vi "DynamicPersonality.vi"(6 "Pass State\n(inicial)":bool=TRUE, 7 "Pinned":T1={"Attc"="Auto", "Strk"="Auto", "Def"=[], "Strk 2"="Auto"}, 8 "Modo Teste ?":bool, 9 "Qtd Min p/ Stk":dbl=2.0, 10 "our_goalie_id":dbl, 11 "input cluster":T3={"our_robots"=[], "enemy_robots"=[], "balls"=[], "geometry"={"line_width"=0, "field_length"=0, "field_width"=0, "boundary_width"=0, "referee_width"=0, "goal_width"=0, "goal_depth"=0, "goal_wall_width"=0, "center_circle_radius"=0, "defense_radius"=0, "defense_stretch"=0, "free_kick_from_defense_dist"=0, "penalty_spot_from_field_line_dist"=0, "penalty_line_from_spot_dist"=0}, "IA Judge"={"stage"="", "command"="", "our_goalie_id"=0.0, "enemy_goalie_id"=0.0, "command enum"=enum."Halt", "Time"=enum."Azul"}, "Received Timestamp"=timestamp(0 s since 1904-01-01), "Events"={"Touch"=FALSE, "Ball out"=FALSE, "id touch"=0.0, "Ball out of \nVision"=FALSE, "Ball inside \nGoalie area"=FALSE, "Robot not responding"=FALSE, "Robots responding status"=[1.0, 1.0, 1.0, 1.0, 1.0, 1.0], "Enemy Ball \nPossession"=FALSE, "Pass State"=FALSE, "id end of pass"=0.0, "Kick"=FALSE, "Id ini Possession"=0.0, "Ball Possesion"=FALSE, "Id Possesion"=0.0, "Direct Kick"=FALSE, "2nd Strk Ativo"=FALSE}}) -> (2 "output cluster":T3={"our_robots"=[], "enemy_robots"=[], "balls"=[], "geometry"={"line_width"=0, "field_length"=0, "field_width"=0, "boundary_width"=0, "referee_width"=0, "goal_width"=0, "goal_depth"=0, "goal_wall_width"=0, "center_circle_radius"=0, "defense_radius"=0, "defense_stretch"=0, "free_kick_from_defense_dist"=0, "penalty_spot_from_field_line_dist"=0, "penalty_line_from_spot_dist"=0}, "IA Judge"={"stage"="", "command"="", "our_goalie_id"=0.0, "enemy_goalie_id"=0.0, "command enum"=enum."Halt", "Time"=enum."Azul"}, "Received Timestamp"=timestamp(0 s since 1904-01-01), "Events"={"Touch"=FALSE, "Ball out"=FALSE, "id touch"=0.0, "Ball out of \nVision"=FALSE, "Ball inside \nGoalie area"=FALSE, "Robot not responding"=FALSE, "Robots responding status"=[1.0, 1.0, 1.0, 1.0, 1.0, 1.0], "Enemy Ball \nPossession"=FALSE, "Pass State"=FALSE, "id end of pass"=0.0, "Kick"=FALSE, "Id ini Possession"=0.0, "Ball Possesion"=FALSE, "Id Possesion"=0.0, "Direct Kick"=FALSE, "2nd Strk Ativo"=FALSE}})   [LabVIEW 2017]
uses:
  Core/AI Input.ctl
  Core/AI Robot.ctl
  Intel/Functions Enum.ctl
  Intel/AttackerStates.ctl
  Path Planning/RRT/PathDests.ctl
  Path Planning/RRT/PathDest.ctl
  Core/AI Ball.ctl
  Core/Field Size.ctl
  Core/AI Judge.ctl
  Intel/Command Enum.ctl
  Util/Events/Events.ctl
  Select Personalitys.ctl
  Util/Select Auto None or Robot.ctl
panel:
  out "Id 2nd Striker\nPinned":u32
  out "2nd Striker\nPinned?":bool=TRUE
  out "Dfdr\nPinned?":bool
  out "Strk\nPinned?":bool
  out "Attck\nPinned?":bool
  in  "Ids validos":u32[](array[numeric])=[42, 42, 42, 42, 42, 42, 42]
  out "Maior prioridade de \natacante é o mais\nproximo da bola?":bool
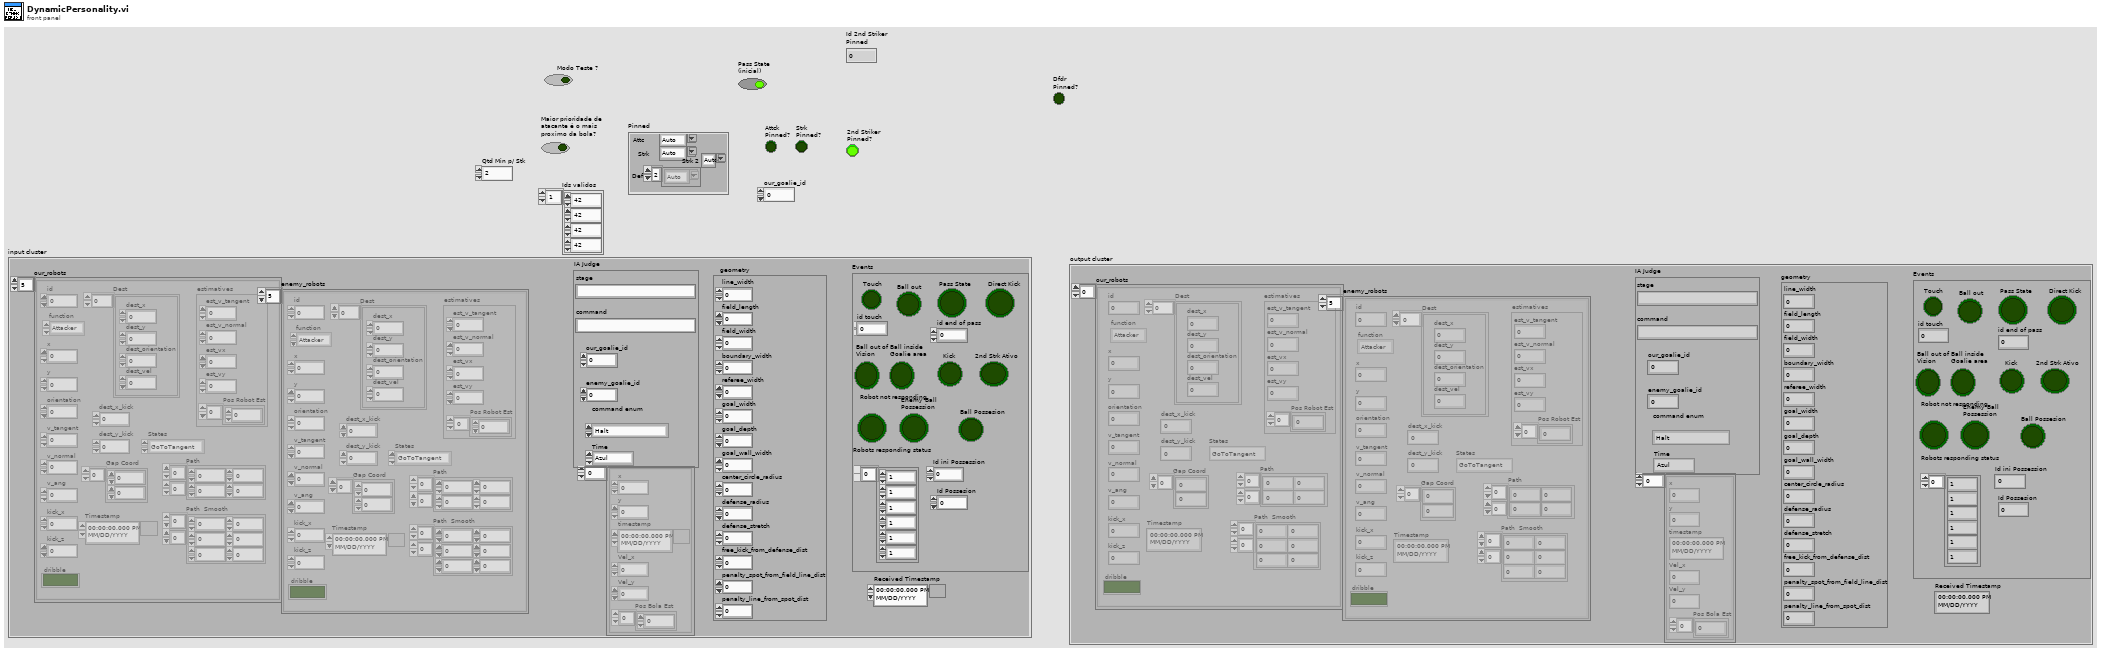
[diagram p1: front panel]
types:
  T1 = typedef "Select Personalitys.ctl" = cluster{"Attc":T2, "Strk":T2, "Def":T2[], "Strk 2":T2}
  T2 = typedef "Select Auto None or Robot.ctl" = string
  T3 = typedef "AI Input.ctl" = cluster{"our_robots":T4[], "enemy_robots":T4[], "balls":T9[], "geometry":T10, "IA Judge":T11, "Received Timestamp":timestamp, "Events":T13}
  T4 = typedef "AI Robot.ctl" = cluster{"id":u32, "function":T5, "x":dbl, "y":dbl, "orientation":dbl, "v_tangent":dbl, "v_normal":dbl, "v_ang":dbl, "kick_x":dbl, "kick_z":dbl, "dribble":bool, "Timestamp":timestamp, "estimatives":cluster{"est_v_tangent":dbl, "est_v_normal":dbl, "est_vx":dbl, "est_vy":dbl, "Pos Robot Est":dbl[]}, "dest_x_kick":dbl, "dest_y_kick":dbl, "Gap Coord":dbl[], "States":T6, "Path ":dbl[][], "Path  Smooth":dbl[][], "Dest":T7}
  T5 = typedef "Functions Enum.ctl" = enum16{"2nd Striker", "Attacker", "Goalie", "Defender", "Striker", "Goto 0", "Dummy", "Kicker", "ZigZag 0", "ZigZag 1", "ZigZag 2", "ZigZag 3", "ZigZag 4", "ZigZag 5", "ZigZag 6", "ZigZag 7", "ZigZag 8", ""}
  T6 = typedef "AttackerStates.ctl" = enum16{"Pass", "GoToTangent", "BallGetting", "GoToKick", ""}
  T7 = typedef "PathDests.ctl" = T8[]
  T8 = typedef "PathDest.ctl" = cluster{"dest_x":dbl, "dest_y":dbl, "dest_orientation":dbl, "dest_vel":dbl}
  T9 = typedef "AI Ball.ctl" = cluster{"x":dbl, "y":dbl, "timestamp":timestamp, "Vel_x":dbl, "Vel_y":dbl, "Pos Bola Est":dbl[]}
  T10 = typedef "Field Size.ctl" = cluster{"line_width":u32, "field_length":u32, "field_width":u32, "boundary_width":u32, "referee_width":u32, "goal_width":u32, "goal_depth":u32, "goal_wall_width":u32, "center_circle_radius":u32, "defense_radius":u32, "defense_stretch":u32, "free_kick_from_defense_dist":u32, "penalty_spot_from_field_line_dist":u32, "penalty_line_from_spot_dist":u32}
  T11 = typedef "AI Judge.ctl" = cluster{"stage":string, "command":string, "our_goalie_id":dbl, "enemy_goalie_id":dbl, "command enum":T12, "Time":enum16{"Azul", "Amarelo"}}
  T12 = typedef "Command Enum.ctl" = enum16{"Halt", "Stop", "Force Start", "PKA Normal Start", "Prepare Kickoff Ally", "PKE Normal Start", "Prepare Kickoff Enemy", "Prepare Penalty Ally", "PPA Normal Start", "Prepare Penalty Enemy", "PPE Normal Start", "Direct Free Enemy", "Direct Free Ally", "Indirect Free Enemy", "Indirect Free Ally", "Timeout Enemy", "Timeout Ally", "Goal Enemy", "Goal Ally", "Ball Placement Enemy", "Ball Placement Ally", "Normal Half Time", "Extra Time Break", "Extra Half Time", "None", "Post Game"}
  T13 = typedef "Events.ctl" = cluster{"Touch":bool, "Ball out":bool, "id touch":dbl, "Ball out of \nVision":bool, "Ball inside \nGoalie area":bool, "Robot not responding":bool, "Robots responding status":dbl[], "Enemy Ball \nPossession":bool, "Pass State":bool, "id end of pass":dbl, "Kick":bool, "Id ini Possession":dbl, "Ball Possesion":bool, "Id Possesion":dbl, "Direct Kick":bool, "2nd Strk Ativo":bool}
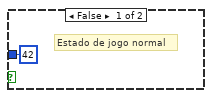
[diagram p4: hidden frame]
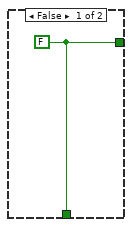
[diagram p9: hidden frame]
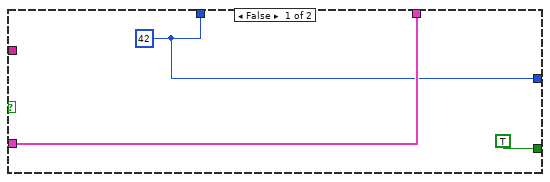
[diagram p11: hidden frame]
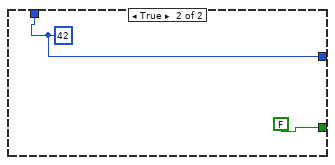
[diagram p13: hidden frame]
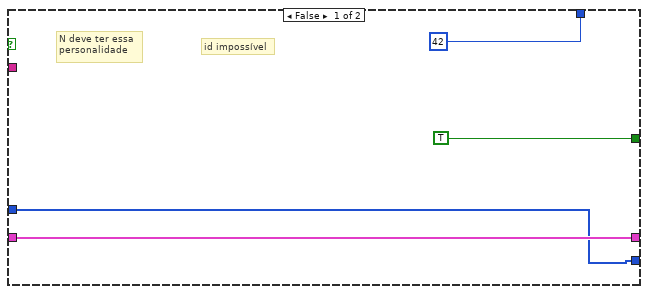
[diagram p17: hidden frame]
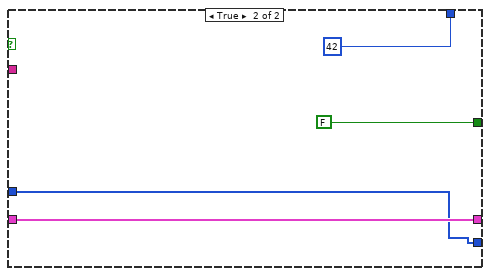
[diagram p19: hidden frame]
diagram:
  # "True: Travado com None\nFalse: Não travado ou travado com id válido"
  # "Descobre id do Striker antes de entrar\nno evento de passe."
  # "personalidades atualizadas"
  # "vai pro feedback node"
  # "personalidades atualizadas"
  # "personalidades atualizadas"
  # "Pinned"
  # "bola parada ?"
  n1 = Unbundle By Name("input cluster") -> ("our_robots"=w148:T4[], "balls"=w105:T9[])
  n2 = Unbundle By Name("Pinned") -> ("Strk"=w149:T2)
  n3 = Not Equal?(x=T2 "None", y=w149) -> (x != y?=w11:bool)
  n4 = case shown="False" w11 {
    tunnel: w149 -> [_ w158]
    tunnel: w148 -> [w153 w157]
    tunnel: [w153 w156] -> w125
    tunnel: [TRUE w155] -> w129
    tunnel: [u32 42 ("Id Maior\nprioridade\natacante") w154] -> w143
    frame False {
      # "id impossível"
      # "N deve ter essa \npersonalidade"
    }
    frame True {
      n5 = Equal?(x=T2 "Auto", y=w158) -> (x = y?=w159:bool)
      n6 = case shown="False" w159 {
        tunnel: w158 -> [w165 _]
        tunnel: w157 -> [w164 w177]
        tunnel: [w163 w177] -> w156
        tunnel: [TRUE FALSE] -> w155
        tunnel: [w161 42] -> w154
        frame False {
          n7 = Decimal String To Number(string=w165) -> (number=w161:i32)  [unwired: 2 in, 1 out]
          n8 = for {
            tunnel: w164 -> [w168] mode=indexing
            tunnel: w161 -> [w169]
            tunnel: [w167] -> w163 mode=indexing
            n9 = Unbundle By Name(w168) -> ("id"=w170:u32)
            n10 = Equal?(x=w169, y=w170) -> (x = y?=w166:bool)
            n11 = case shown="True" w166 {
              tunnel: w168 -> [w171 w174]
              tunnel: [w171 w173] -> w167
              frame False {
              }
              frame True {
                n12 = Bundle By Name(cluster=w174, "function"=Functions_Enum."Striker") -> (w173:T4)
              }
            }
          }
        }
        frame True {
        }
      }
    }
  }
  "Strk\nPinned?" <- w129
  n13 = Unbundle By Name("Pinned") -> ("Def"=w127:T2[])
  n14 = for {
    tunnel: w127 -> [w186] mode=indexing
    tunnel: [w183] -> w123 mode=indexing
    shift-right: [w184] -> w124
    shift-left: w125 -> [w185]
    shift-right: [w181] -> w126
    shift-left: FALSE -> [w182]
    shift-right: [w178] -> _
    shift-left: i32[] [] -> [w179]
    n15 = Not Equal?(x=T2 "None", y=w186) -> (x != y?=w187:bool)
    n16 = case shown="True" w187 {
      tunnel: w186 -> [_ w201]
      tunnel: w185 -> [w192 w200]
      tunnel: [w192 w199] -> w184
      tunnel: [TRUE w198] -> w180
      tunnel: [u32 42 ("Id Maior\nprioridade\natacante") w197] -> w183
      tunnel: w179 -> [w191 w196]
      tunnel: [w191 w195] -> w178
      frame False {
        # "id impossível"
        # "N deve ter essa \npersonalidade"
      }
      frame True {
        n17 = Equal?(x=T2 "Auto", y=w201) -> (x = y?=w202:bool)
        n18 = case shown="False" w202 {
          tunnel: w201 -> [w210 _]
          tunnel: w200 -> [w209 w229]
          tunnel: [w208 w229] -> w199
          tunnel: [TRUE FALSE] -> w198
          tunnel: [w206 42] -> w197
          tunnel: w196 -> [w205 w226]
          tunnel: [w204 w226] -> w195
          frame False {
            n19 = Decimal String To Number(string=w210) -> (number=w206:i32)  [unwired: 2 in, 1 out]
            n20 = for {
              tunnel: w209 -> [w216] mode=indexing
              tunnel: w206 -> [w217]
              tunnel: [w215] -> w208 mode=indexing
              tunnel: w205 -> [w212]
              tunnel: [w211] -> w204
              n21 = Unbundle By Name(w216) -> ("id"=w213:u32)
              n22 = Equal?(x=w217, y=w213) -> (x = y?=w214:bool)
              n23 = case shown="True" w214 {
                tunnel: w216 -> [w219 w225]
                tunnel: [w219 w224] -> w215
                tunnel: w213 -> [_ w221]
                tunnel: w212 -> [w218 w222]
                tunnel: [w218 w220] -> w211
                frame False {
                }
                frame True {
                  n24 = Bundle By Name(cluster=w225, "function"=Functions_Enum."Defender") -> (w224:T4)
                  n25 = Insert Into Array(array=w222, new element=w221) -> (w220:i32[])  [unwired: 1 in]
                }
              }
            }
          }
          frame True {
          }
        }
      }
    }
    n26 = case shown="True" w182 {
      tunnel: [w189 TRUE] -> w181
      tunnel: w180 -> [w189 _]
      frame False {
      }
      frame True {
      }
    }
  }
  "Dfdr\nPinned?" <- w126
  n27 = Unbundle By Name("Pinned") -> ("Attc"=w146:T2)
  n28 = Not Equal?(x=T2 "None", y=w146) -> (x != y?=w145:bool)
  n29 = case shown="True" w145 {
    tunnel: w146 -> [_ w237]
    tunnel: w124 -> [w232 w236]
    tunnel: [w232 w235] -> w50
    tunnel: [TRUE w234] -> w128
    tunnel: [42 w233] -> w144
    frame False {
      # "id impossível"
      # "N deve ter essa \npersonalidade"
    }
    frame True {
      n30 = Equal?(x=T2 "Auto", y=w237) -> (x = y?=w238:bool)
      n31 = case shown="False" w238 {
        tunnel: w237 -> [w244 _]
        tunnel: w236 -> [w243 w256]
        tunnel: [w242 w256] -> w235
        tunnel: [TRUE FALSE] -> w234
        tunnel: [w240 42] -> w233
        frame False {
          n32 = Decimal String To Number(string=w244) -> (number=w240:i32)  [unwired: 2 in, 1 out]
          n33 = for {
            tunnel: w243 -> [w247] mode=indexing
            tunnel: w240 -> [w248]
            tunnel: [w246] -> w242 mode=indexing
            n34 = Unbundle By Name(w247) -> ("id"=w249:u32)
            n35 = Equal?(x=w248, y=w249) -> (x = y?=w245:bool)
            n36 = case shown="True" w245 {
              tunnel: w247 -> [w250 w253]
              tunnel: [w250 w252] -> w246
              frame False {
              }
              frame True {
                n37 = Bundle By Name(cluster=w253, "function"=Functions_Enum."Attacker") -> (w252:T4)
              }
            }
          }
        }
        frame True {
        }
      }
    }
  }
  "Attck\nPinned?" <- w128
  n38 = Unbundle By Name("Pinned") -> ("Strk 2"=w51:T2)
  n39 = Not Equal?(x=w51, y=T2 "None" ("Strk 2")) -> (x != y?=w53:bool)
  n40 = case shown="True" w53 {
    tunnel: [w257 w263] -> w22
    tunnel: [TRUE w262] -> w52
    tunnel: w51 -> [_ w264]
    tunnel: w50 -> [w258 w261]
    tunnel: [w258 w261] -> w41
    tunnel: [w257 w260] -> w21
    frame False {
      w257 = u32 42
    }
    frame True {
      n41 = Equal?(x=w264, y=T2 "Auto" ("Strk 2")) -> (x = y?=w265:bool)
      n42 = case shown="False" w265 {
        tunnel: w264 -> [w271 _]
        tunnel: [w268 w280] -> w263
        tunnel: [TRUE FALSE] -> w262
        tunnel: w261 -> [w269 _]
        tunnel: [w267 w280] -> w260
        frame False {
          n43 = Decimal String To Number(string=w271) -> (number=w268:i32)  [unwired: 2 in, 1 out]
          n44 = for {
            tunnel: w269 -> [w276] mode=indexing
            tunnel: w268 -> [w277]
            shift-right: [w274] -> w267
            shift-left: _ -> [w272]
            n45 = Unbundle By Name(w276) -> ("id"=w273:u32)
            n46 = Equal?(x=w277, y=w273) -> (x = y?=w275:bool)
            n47 = case shown="True" w275 {
              tunnel: [w278 w279] -> w274
              tunnel: w273 -> [_ w279]
              tunnel: w272 -> [w278 _]
              frame False {
              }
              frame True {
              }
            }
          }
        }
        frame True {
          w280 = u32 42
        }
      }
    }
  }
  "2nd Striker\nPinned?" <- w52
  "Id 2nd Striker\nPinned" <- w21
  n48 = for {
    tunnel: w41 -> [w295] mode=indexing
    tunnel: w144 -> [w294]
    tunnel: w143 -> [w293]
    tunnel: w123 -> [w287]
    shift-right: [w290] -> w141
    shift-left: u32[] [] -> [w291]
    tunnel: u32 42 -> [w284]
    # "Deve ter striker?"
    # "Deve ter atacante?"
    n49 = Unbundle By Name(w295) -> ("id"=w283:u32)
    n50 = for {
      tunnel: w283 -> [w298]
      tunnel: [w297] -> w285 mode=indexing
      tunnel: w287 -> [w296] mode=indexing
      n51 = Equal?(x=w296, y=w298) -> (x = y?=w297:bool)
    }
    n52 = Equal?(x=w294, y=w283) -> (x = y?=w292:bool)
    n53 = Equal?(x=w293, y=w283) -> (x = y?=w289:bool)
    n54 = Or Array Elements(Boolean array=w285) -> (logical OR=w286:bool)
    n55 = Equal?(x=w284, y=w283) -> (x = y?=w282:bool)
    n56 = Compound Arithmetic op=OR(w289, w286, w292, w282) -> (w288:bool)
    n57 = case shown="False" w288 {
      tunnel: [w299 w302] -> w290
      tunnel: w291 -> [w301 w302]
      tunnel: w283 -> [w300 _]
      frame False {
        n58 = Insert Into Array(array=w301, new element=w300) -> (w299:u32[])  [unwired: 1 in]
      }
      frame True {
      }
    }
  }
  n59 = Reverse 1D Array(array=w141) -> (reversed array=w139:u32[])
  n60 = for {
    tunnel: w139 -> [w307] mode=indexing
    tunnel: "our_goalie_id" -> [w306]
    shift-right: [w303] -> w60
    shift-left: w139 -> [w305]
    i -> [w304]
    n61 = Equal?(x=w307, y=w306) -> (x = y?=w308:bool)
    n62 = case shown="True" w308 {
      tunnel: w305 -> [w309 w312]
      tunnel: w304 -> [_ w311]
      tunnel: [w309 w310] -> w303
      frame False {
      }
      frame True {
        n63 = Delete From Array(array=w312, index=w311) -> (array with subset deleted=w310:u32[])  [unwired: 1 in, 1 out]
      }
    }
  }
  n64 = Unbundle By Name("input cluster") -> ("Events.Pass State"=w23:bool, "Events.Touch"=w45:bool)
  n65 = case shown="True" w23 {
    tunnel: [u32 42 w314] -> _
    tunnel: w22 -> [_ w314]
    frame False {
      # "Estado de jogo normal"
    }
    frame True {
      # "Evento de passe"
    }
  }
  n66 = Unbundle By Name("input cluster") -> ("balls"=w138:T9[])  [unwired: 1 out]
  n67 = Index Array(array=w138) -> (element=w61:T9)  [unwired: 1 in]
  n68 = for {
    tunnel: w61 -> [w323]
    tunnel: w60 -> [w316] mode=indexing
    tunnel: w41 -> [w326]
    shift-right: [w320] -> w136
    shift-left: dbl[] [] -> [w319]
    shift-right: [w317] -> _
    shift-left: 0.0 -> [w318]
    n69 = while {
      tunnel: w326 -> [w332] mode=indexing
      tunnel: [w331] -> w325
      tunnel: [w330] -> w324
      tunnel: w316 -> [w329]
      tunnel: [w327] -> w315
      stop <- w327 stop-if-true
      n70 = Unbundle By Name(w332) -> ("id"=w328:u32, "x"=w331:dbl, "y"=w330:dbl)
      n71 = Equal?(x=w329, y=w328) -> (x = y?=w327:bool)
    }
    n72 = Unbundle By Name(w323) -> ("x"=w322:dbl, "y"=w321:dbl)
    n73 = case shown="True" w315 {
      tunnel: w325 -> [_ w345]
      tunnel: w324 -> [_ w343]
      tunnel: w322 -> [_ w346]
      tunnel: w321 -> [_ w344]
      tunnel: [w334 w339] -> w320
      tunnel: w319 -> [w334 w338]
      tunnel: w318 -> [w333 w336]
      tunnel: [w333 w335] -> w317
      frame False {
      }
      frame True {
        n74 = Subtract(x=w346, y=w345) -> (x-y=w342:dbl)
        n75 = Subtract(x=w344, y=w343) -> (x-y=w341:dbl)
        n76 = Build Array(w342, w341) -> (w340:dbl[])
        n77 = call "Modulo.vi"("2D vector"=w340) -> ("Modulo"=w337:dbl)  [unwired: 10 in]
        n78 = Insert Into Array(array=w338, index=w336, new element=w337) -> (w339:dbl[])
        n79 = Increment(x=w336) -> (x+1=w335:dbl)
      }
    }
  }
  n80 = feedback #1(FALSE) -> (w46:bool)
  n81 = Index Array(array=w136) -> (element #1=w134:dbl, element #2=w135:dbl)  [unwired: 2 in]
  n82 = feedback #2() -> (w42:bool)  [unwired: 1 in]
  n83 = case shown="True" w23 {
    tunnel: [w347 w350] -> w44
    tunnel: [w347 w349] -> w48
    tunnel: w46 -> [_ w351]
    tunnel: w45 -> [_ w352]
    tunnel: w42 -> [_ w348]
    frame False {
      w347 = FALSE
    }
    frame True {
      n84 = case shown="True" w352 {
        tunnel: [w353 TRUE] -> w349
        tunnel: w351 -> [w353 _]
        frame False {
        }
        frame True {
        }
      }
      n85 = And(x=w348, y=w349) -> (x .and. y?=w350:bool)
    }
  }
  n86 = feedback-in #1(w48) -> ()
  n87 = Less?(x=w134, y=w135) -> (x < y?=w133:bool)
  "Maior prioridade de \natacante é o mais\nproximo da bola?" <- w133
  n88 = Array Size(array=w41) -> (size(s)=w131:i32)
  n89 = local read "Strk\nPinned?"() -> (w58:bool)
  n90 = local read "Attck\nPinned?"() -> (w59:bool)
  n91 = Greater?(x=w131, y=0) -> (0:w132:bool)
  n92 = local read "Id 2nd Striker\nPinned"() -> (w26:u32)
  n93 = local read "2nd Striker\nPinned?"() -> (w28:bool)
  n94 = Equal?(x=w26, y=u32 42) -> (x = y?=w29:bool)
  n95 = And(x=w29, y=w28) -> (x .and. y?=w27:bool)
  n96 = Not Equal?(x=w26, y=u32 42) -> (x != y?=w24:bool)
  n97 = feedback #3() -> (w122:T4[])  [unwired: 1 in]
  n98 = feedback #4(FALSE ("Kick")) -> (w111:bool)
  n99 = Index Array(array=w105) -> (element=w104:T9)  [unwired: 1 in]
  n100 = Unbundle By Name(w104) -> ("Vel_x"=w74:dbl, "Vel_y"=w72:dbl)
  n101 = Absolute Value(x=w72) -> (abs(x)=w71:dbl)
  n102 = Absolute Value(x=w74) -> (abs(x)=w73:dbl)
  n103 = Less Or Equal?(x=w73, y=0.05) -> (x <= y?=w6:bool)
  n104 = Less Or Equal?(x=w71, y=0.05) -> (x <= y?=w5:bool)
  n105 = feedback #5() -> (w2:bool)  [unwired: 1 in]
  n106 = local read "2nd Striker\nPinned?"() -> (w19:bool)
  n107 = local read "Id 2nd Striker\nPinned"() -> (w15:u32)
  n108 = feedback #6() -> (w40:u32)  [unwired: 1 in]
  n109 = feedback #7() -> (w36:u32)  [unwired: 1 in]
  n110 = Not Equal?(x=u32 42, y=w15) -> (x != y?=w18:bool)
  n111 = And(x=w18, y=w19) -> (x .and. y?=w16:bool)
  n112 = feedback #8(FALSE) -> (w116:bool)
  n113 = for {
    tunnel: w41 -> [w384] mode=indexing
    tunnel: w139 -> [w364]
    tunnel: "our_goalie_id" -> [w390]
    tunnel: [w389] -> w35 mode=indexing
    tunnel: w133 -> [w387]
    tunnel: w132 -> [w386]
    tunnel: "input cluster" -> [w385]
    tunnel: w122 -> [w383]
    tunnel: w116 -> [w379]
    tunnel: "input cluster" -> [w371]
    tunnel: [w370] -> w103
    tunnel: [w368] -> _
    tunnel: w41 -> [w367]
    tunnel: w61 -> [w366]
    tunnel: w60 -> [w365]
    tunnel: w59 -> [w363]
    tunnel: w58 -> [w362]
    tunnel: w27 -> [w361]
    tunnel: w44 -> [w360]
    tunnel: [w355] -> w43
    tunnel: w24 -> [w357]
    tunnel: w21 -> [w356]
    tunnel: [w355] -> w3
    i -> [w382]
    n114 = Unbundle By Name(w385) -> ("Events.Pass State"=w377:bool, "IA Judge.command enum"=w368:T12)
    n115 = Unbundle By Name(w384) -> ("id"=w391:u32)
    n116 = for {
      tunnel: w364 -> [w946] mode=indexing
      tunnel: w391 -> [w947]
      shift-right: [w944] -> w388
      shift-left: FALSE -> [w945]
      n117 = Equal?(x=w946, y=w947) -> (x = y?=w943:bool)
      n118 = case shown="True" w943 {
        tunnel: w945 -> [w948 _]
        tunnel: [w948 TRUE] -> w944
        frame False {
        }
        frame True {
        }
      }
    }
    n119 = feedback-in #9(w377) -> ()
    n120 = feedback #9() -> (w378:bool)  [unwired: 1 in]
    n121 = Equal?(x=w377, y=TRUE) -> (x = y?=w373:bool)
    n122 = Equal?(x=w378, y=FALSE) -> (x = y?=w374:bool)
    n123 = And(x=w374, y=w373) -> (x .and. y?=w372:bool)
    n124 = feedback #10() -> (w380:bool)  [unwired: 1 in]
    n125 = case shown="False" w372 {
      selector: w372 -> [_ w405]
      tunnel: [w397 w405] -> w381
      tunnel: w380 -> [w396 _]
      tunnel: w379 -> [w395 _]
      tunnel: [w394 w405] -> w355
      tunnel: w377 -> [w393 _]
      frame False {
        n126 = case shown="True" w395 {
          tunnel: w393 -> [w401 _]
          tunnel: [w398 w404] -> w397
          tunnel: w396 -> [w400 _]
          tunnel: [w399 w404] -> w394
          frame False {
            n127 = case shown="True" w401 {
              selector: w401 -> [w402 _]
              tunnel: w400 -> [_ w403]
              tunnel: [w402 w403] -> w399
              tunnel: [w402 w403] -> w398
              frame False {
              }
              frame True {
              }
            }
          }
          frame True {
            w404 = FALSE
          }
        }
      }
      frame True {
      }
    }
    n128 = feedback-in #10(w381) -> ()
    n129 = Bundle By Name(cluster=w371, "Events.2nd Strk Ativo"="Pass State\n(inicial)", "Events.Pass State"=w355) -> (w370:T3)
    n130 = Unbundle By Name(w370) -> ("Events.Ball out of \nVision"=w369:bool, "Events.2nd Strk Ativo"=w359:bool)
    n131 = case shown="Default" w368 {
      tunnel: w391 -> [w408 w442 w474]
      tunnel: w390 -> [w406 w443 w473]
      tunnel: w384 -> [w410 w446 w472]
      tunnel: [w411 w445 w471] -> w389
      tunnel: w365 -> [w407 _ w470]
      tunnel: w388 -> [w409 _ w469]
      tunnel: w387 -> [_ _ w468]
      tunnel: w386 -> [_ _ w467]
      tunnel: w383 -> [_ _ w456]
      tunnel: w382 -> [_ _ w466]
      tunnel: w355 -> [_ _ _]
      tunnel: w369 -> [_ _ w458]
      tunnel: w367 -> [_ _ w464]
      tunnel: w366 -> [_ _ w463]
      tunnel: w363 -> [_ _ w462]
      tunnel: w362 -> [_ _ w461]
      tunnel: w361 -> [_ _ w460]
      tunnel: w360 -> [_ _ w459]
      tunnel: w359 -> [_ _ w457]
      tunnel: w357 -> [_ _ w455]
      tunnel: w356 -> [_ _ w454]
      tunnel: w355 -> [_ _ w453]
      frame "Prepare Penalty Ally", "PPA Normal Start" {
        # "um atacante, geral defesa"
        n132 = case shown="True" w409 {
          tunnel: [w412 w418] -> w411
          tunnel: w410 -> [w412 w417]
          tunnel: w408 -> [_ w414]
          tunnel: w407 -> [_ w416]
          tunnel: w406 -> [_ w413]
          frame False {
            # "personalidade já definida"
          }
          frame True {
            # "id válido para personalidade dinâmica"
            n133 = Equal?(x=w413, y=w414) -> (x = y?=w415:bool)
            n134 = case shown="False" w415 {
              tunnel: [w423 w440] -> w418
              tunnel: w417 -> [w422 w439]
              tunnel: w414 -> [w420 _]
              tunnel: w416 -> [w419 _]
              frame False {
                # "n é goleiro"
                n135 = local read "Attck\nPinned?"() -> (w421:bool)
                n136 = case shown="True" w421 {
                  tunnel: [w429 w437] -> w423
                  tunnel: w422 -> [w428 w436]
                  tunnel: w420 -> [w426 _]
                  tunnel: w419 -> [w424 _]
                  frame False {
                    # "atacante n definido"
                    n137 = Index Array(array=w424) -> (element=w425:u32)  [unwired: 1 in]
                    n138 = Equal?(x=w426, y=w425) -> (x = y?=w427:bool)
                    n139 = case shown="True" w427 {
                      tunnel: [w431 w434] -> w429
                      tunnel: w428 -> [w430 w433]
                      frame False {
                        # "n é o maior dos ids válidos"
                        n140 = Bundle By Name(cluster=w430, "function"=Functions_Enum."Defender") -> (w431:T4)
                      }
                      frame True {
                        # "maior dos ids válidos"
                        n141 = Bundle By Name(cluster=w433, "function"=Functions_Enum."Attacker") -> (w434:T4)
                      }
                    }
                  }
                  frame True {
                    # "atacante já definido"
                    n142 = Bundle By Name(cluster=w436, "function"=Functions_Enum."Defender") -> (w437:T4)
                  }
                }
              }
              frame True {
                # "é goleiro"
                n143 = Bundle By Name(cluster=w439, "function"=Functions_Enum."Goalie") -> (w440:T4)
              }
            }
          }
        }
      }
      frame "Prepare Penalty Enemy", "PPE Normal Start" {
        # "geral defesa"
        n144 = Equal?(x=w443, y=w442) -> (x = y?=w444:bool)
        n145 = case shown="False" w444 {
          tunnel: w446 -> [w449 w452]
          tunnel: [w448 w451] -> w445
          frame True {
            # "é goleiro"
            n146 = Bundle By Name(cluster=w449, "function"=Functions_Enum."Goalie") -> (w448:T4)
          }
          frame False {
            # "n é goleiro"
            n147 = Bundle By Name(cluster=w452, "function"=Functions_Enum."Defender") -> (w451:T4)
          }
        }
      }
      frame Default {
        n148 = Or(x=w458, y=w457) -> (x .or. y?=w465:bool)
        n149 = case shown="True" w465 {
          tunnel: w474 -> [w484 _]
          tunnel: w473 -> [w483 w623]
          tunnel: w472 -> [w482 w617]
          tunnel: [w481 w626] -> w471
          tunnel: w470 -> [w480 w618]
          tunnel: w469 -> [w479 w625]
          tunnel: w468 -> [w478 _]
          tunnel: w467 -> [w477 w621]
          tunnel: w456 -> [_ w614]
          tunnel: w466 -> [_ w613]
          tunnel: w464 -> [_ w627]
          tunnel: w463 -> [_ w628]
          tunnel: w462 -> [w476 w619]
          tunnel: w461 -> [w475 w620]
          tunnel: w460 -> [_ w622]
          tunnel: w459 -> [_ w615]
          tunnel: w455 -> [_ w612]
          tunnel: w454 -> [_ w611]
          tunnel: w453 -> [_ w610]
          frame False {
            # "estado de jogo normal"
            n150 = case shown="True" w479 {
              tunnel: w484 -> [_ w491]
              tunnel: w483 -> [_ w495]
              tunnel: w482 -> [w485 w493]
              tunnel: [w485 w492] -> w481
              tunnel: w480 -> [_ w490]
              tunnel: w478 -> [_ w489]
              tunnel: w477 -> [_ w488]
              tunnel: w476 -> [_ w487]
              tunnel: w475 -> [_ w486]
              frame False {
                # "Personalidade já definida"
              }
              frame True {
                # "Id válido para personalidade dinâmica"
                n151 = Equal?(x=w495, y=w491) -> (x = y?=w494:bool)
                n152 = case shown="False" w494 {
                  tunnel: w493 -> [w502 w608]
                  tunnel: [w503 w607] -> w492
                  tunnel: w491 -> [w500 _]
                  tunnel: w490 -> [w501 _]
                  tunnel: w489 -> [w499 _]
                  tunnel: w488 -> [w498 _]
                  tunnel: w487 -> [w497 _]
                  tunnel: w486 -> [w496 _]
                  frame False {
                    # "n é goleiro"
                    n153 = Index Array(array=w501) -> (element=w504:u32)  [unwired: 1 in]
                    n154 = Equal?(x=w500, y=w504) -> (x = y?=w505:bool)
                    n155 = case shown="True" w505 {
                      tunnel: [w510 w566] -> w503
                      tunnel: w502 -> [w511 w565]
                      tunnel: w501 -> [w512 _]
                      tunnel: w500 -> [w509 _]
                      tunnel: w499 -> [w507 w564]
                      tunnel: w498 -> [w506 w563]
                      tunnel: w497 -> [_ w562]
                      tunnel: w496 -> [_ w561]
                      frame False {
                        # "n é o maior id dos válidos"
                        n156 = Index Array(array=w512) -> (element #2=w508:u32)  [unwired: 2 in, 1 out]
                        n157 = Equal?(x=w509, y=w508) -> (x = y?=w513:bool)
                        n158 = case shown="True" w513 {
                          tunnel: w511 -> [w514 w520]
                          tunnel: [w515 w519] -> w510
                          tunnel: w507 -> [_ w518]
                          tunnel: w506 -> [_ w517]
                          frame False {
                            # "n é o segundo maior id"
                            n159 = Bundle By Name(cluster=w514, "function"=Functions_Enum."Defender") -> (w515:T4)
                          }
                          frame True {
                            # "segundo maior id"
                            n160 = local read "Strk\nPinned?"() -> (w521:bool)
                            n161 = case shown="False" w521 {
                              tunnel: w520 -> [w525 w553]
                              tunnel: [w526 w552] -> w519
                              tunnel: w518 -> [w523 _]
                              tunnel: w517 -> [w522 _]
                              frame False {
                                # "striker n definido"
                                n162 = local read "Attck\nPinned?"() -> (w524:bool)
                                n163 = case shown="False" w524 {
                                tunnel: [w530 w550] -> w526
                                tunnel: w525 -> [w529 w549]
                                tunnel: w523 -> [w528 _]
                                tunnel: w522 -> [w527 _]
                                frame False {
                                # "attacker ainda n definido"
                                n164 = case shown="True" w528 {
                                tunnel: [w533 w542] -> w530
                                tunnel: w529 -> [w532 w541]
                                tunnel: w527 -> [w531 w540]
                                frame False {
                                # "mais perto da bola"
                                n165 = case shown="True" w531 {
                                tunnel: [w535 w538] -> w533
                                tunnel: w532 -> [w534 w537]
                                frame True {
                                n166 = Bundle By Name(cluster=w534, "function"=Functions_Enum."Attacker") -> (w535:T4)
                                }
                                frame False {
                                n167 = Bundle By Name(cluster=w537, "function"=Functions_Enum."Defender") -> (w538:T4)
                                }
                                }
                                }
                                frame True {
                                # "mais longe da bola"
                                n168 = case shown="False" w540 {
                                tunnel: [w544 w547] -> w542
                                tunnel: w541 -> [w543 w546]
                                frame True {
                                n169 = Bundle By Name(cluster=w543, "function"=Functions_Enum."Striker") -> (w544:T4)
                                }
                                frame False {
                                n170 = Bundle By Name(cluster=w546, "function"=Functions_Enum."Defender") -> (w547:T4)
                                }
                                }
                                }
                                }
                                }
                                frame True {
                                # "attacker travado"
                                n171 = Bundle By Name(cluster=w549, "function"=Functions_Enum."Defender") -> (w550:T4)
                                }
                                }
                              }
                              frame True {
                                # "striker travado"
                                n172 = local read "Attck\nPinned?"() -> (w554:bool)
                                n173 = case shown="False" w554 {
                                tunnel: w553 -> [w555 w558]
                                tunnel: [w556 w559] -> w552
                                frame False {
                                # "atacante n definido"
                                n174 = Bundle By Name(cluster=w555, "function"=Functions_Enum."Defender") -> (w556:T4)
                                }
                                frame True {
                                # "atacante travado"
                                n175 = Bundle By Name(cluster=w558, "function"=Functions_Enum."Defender") -> (w559:T4)
                                }
                                }
                              }
                            }
                          }
                        }
                      }
                      frame True {
                        # "maior id dos válidos"
                        n176 = case shown="True" w562 {
                          tunnel: [w571 w593] -> w566
                          tunnel: w565 -> [w570 w592]
                          tunnel: w564 -> [w569 _]
                          tunnel: w563 -> [w568 w591]
                          tunnel: w561 -> [w567 _]
                          frame False {
                            # "Atacante ainda n definido"
                            n177 = case shown="True" w569 {
                              tunnel: [w575 w589] -> w571
                              tunnel: w570 -> [w574 w588]
                              tunnel: w568 -> [w573 _]
                              tunnel: w567 -> [w572 _]
                              frame False {
                                # "n é o mais perto da bola"
                                n178 = case shown="True" w572 {
                                tunnel: [w578 w586] -> w575
                                tunnel: w574 -> [w577 w585]
                                tunnel: w573 -> [w576 _]
                                frame False {
                                n179 = case shown="False" w576 {
                                tunnel: [w580 w583] -> w578
                                tunnel: w577 -> [w579 w582]
                                frame True {
                                n180 = Bundle By Name(cluster=w579, "function"=Functions_Enum."Striker") -> (w580:T4)
                                }
                                frame False {
                                n181 = Bundle By Name(cluster=w582, "function"=Functions_Enum."Attacker") -> (w583:T4)
                                }
                                }
                                }
                                frame True {
                                n182 = Bundle By Name(cluster=w585, "function"=Functions_Enum."Attacker") -> (w586:T4)
                                }
                                }
                              }
                              frame True {
                                # "mais perto da bola"
                                n183 = Bundle By Name(cluster=w588, "function"=Functions_Enum."Attacker") -> (w589:T4)
                              }
                            }
                          }
                          frame True {
                            # "Atacande já travado"
                            n184 = local read "Strk\nPinned?"() -> (w594:bool)
                            n185 = case shown="False" w594 {
                              tunnel: [w597 w605] -> w593
                              tunnel: w592 -> [w596 w604]
                              tunnel: w591 -> [w595 _]
                              frame False {
                                # "Striker ainda n definido"
                                n186 = case shown="False" w595 {
                                tunnel: [w599 w602] -> w597
                                tunnel: w596 -> [w598 w601]
                                frame True {
                                n187 = Bundle By Name(cluster=w598, "function"=Functions_Enum."Striker") -> (w599:T4)
                                }
                                frame False {
                                n188 = Bundle By Name(cluster=w601, "function"=Functions_Enum."Defender") -> (w602:T4)
                                }
                                }
                              }
                              frame True {
                                # "Sobra defesa"
                                # "Striker já travado"
                                n189 = Bundle By Name(cluster=w604, "function"=Functions_Enum."Defender") -> (w605:T4)
                              }
                            }
                          }
                        }
                      }
                    }
                  }
                  frame True {
                    # "é goleiro"
                    n190 = Bundle By Name(cluster=w608, "function"=Functions_Enum."Goalie") -> (w607:T4)
                  }
                }
              }
            }
          }
          frame True {
            # "2nd Striker Ativo"
            n191 = case shown="False" w615 {
              tunnel: w628 -> [w651 _]
              tunnel: w627 -> [w650 _]
              tunnel: w625 -> [w646 _]
              tunnel: w617 -> [w645 _]
              tunnel: [w644 w938] -> w624
              tunnel: w623 -> [w642 _]
              tunnel: w622 -> [w639 _]
              tunnel: w621 -> [w638 _]
              tunnel: w620 -> [w637 _]
              tunnel: w619 -> [w636 _]
              tunnel: w618 -> [w634 _]
              tunnel: w617 -> [w633 w942]
              tunnel: [w633 w942] -> w616
              tunnel: w614 -> [_ w941]
              tunnel: w613 -> [_ w940]
              tunnel: w612 -> [w632 _]
              tunnel: w611 -> [w631 _]
              tunnel: w610 -> [w629 _]
              frame False {
                (unwired) 5 ("y")
                w649 = inf
                # "Após ter iniciado o evento passe,\nattacker ainda não tocou a bola\n                        OU\nAttacker já tocou a bola e já \nacabou pass state."
                n192 = Array Size(array=w650) -> (size(s)=w647:i32)
                n193 = Greater Or Equal?(x=w647, y=0) -> (x >= y?=w641:bool)
                n194 = Build Array(w649, w649) -> (w648:dbl[])
                n195 = Unbundle By Name(w645) -> ("id"=w643:u32)
                n196 = for {
                  tunnel: w650 -> [w908] mode=indexing
                  tunnel: w651 -> [w902]
                  shift-right: [w898] -> w640
                  shift-left: w648 -> [w899]
                  tunnel: w642 -> [w903]
                  tunnel: w634 -> [w897]
                  n197 = Unbundle By Name(w908) -> ("id"=w896:u32, "x"=w907:dbl, "y"=w906:dbl)
                  n198 = Unbundle By Name(w902) -> ("x"=w905:dbl, "y"=w904:dbl)
                  n199 = for {
                    tunnel: w897 -> [w913] mode=indexing
                    tunnel: w896 -> [w912]
                    shift-right: [w910] -> w894
                    shift-left: FALSE -> [w909]
                    n200 = Equal?(x=w913, y=w912) -> (x = y?=w911:bool)
                    n201 = case shown="True" w909 {
                      tunnel: [w914 TRUE] -> w910
                      tunnel: w911 -> [w914 _]
                      frame False {
                      }
                      frame True {
                      }
                    }
                  }
                  n202 = Build Array(w907, w906) -> (w900:dbl[])
                  n203 = Build Array(w905, w904) -> (w901:dbl[])
                  n204 = case shown="True" w894 {
                    tunnel: w903 -> [_ w923]
                    tunnel: w901 -> [_ w921]
                    tunnel: w900 -> [_ w920]
                    tunnel: w899 -> [w916 w919]
                    tunnel: [w916 w918] -> w898
                    tunnel: w896 -> [_ w917]
                    frame False {
                      # "Robô que está passadno\nno código é um dos fixados\nno pinned"
                    }
                    frame True {
                      # "Robô que está passando\nno código é um dos permitidos\np/ personalidade dinâmica"
                      n205 = Equal?(x=w917, y=w923) -> (x = y?=w922:bool)
                      n206 = case shown="False" w922 {
                        tunnel: w921 -> [w932 _]
                        tunnel: w920 -> [w931 _]
                        tunnel: w919 -> [w926 w937]
                        tunnel: w917 -> [w928 _]
                        tunnel: [w927 w937] -> w918
                        frame False {
                          n207 = Subtract(x=w932, y=w931) -> (x-y=w930:dbl[])
                          n208 = Index Array(array=w926) -> (element #2=w924:dbl)  [unwired: 2 in, 1 out]
                          n209 = call "Modulo.vi"("2D vector"=w930) -> ("Modulo"=w925:dbl)  [unwired: 10 in]
                          n210 = Greater?(x=w924, y=w925) -> (0:w929:bool)
                          n211 = case shown="True" w929 {
                            tunnel: w925 -> [_ w936]
                            tunnel: w928 -> [_ w935]
                            tunnel: [w933 w934] -> w927
                            tunnel: w926 -> [w933 _]
                            frame False {
                            }
                            frame True {
                              n212 = Build Array(w935, w936) -> (w934:dbl[])
                            }
                          }
                        }
                        frame True {
                        }
                      }
                    }
                  }
                }
                n213 = case shown="False" w636 {
                  tunnel: w640 -> [w654 _]
                  tunnel: w634 -> [w653 w667]
                  tunnel: [w652 w667] -> w635
                  frame False {
                    # "Attacker ainda não definido"
                    n214 = for {
                      tunnel: w653 -> [w662] mode=indexing
                      tunnel: w654 -> [w661]
                      tunnel: w653 -> [w658]
                      shift-right: [w656] -> w652
                      shift-left: _ -> [w655]
                      i -> [w657]
                      n215 = Index Array(array=w661) -> (element=w660:dbl)  [unwired: 1 in]
                      n216 = Equal?(x=w660, y=w662) -> (x = y?=w659:bool)
                      n217 = case shown="True" w659 {
                        tunnel: w658 -> [_ w666]
                        tunnel: w657 -> [_ w665]
                        tunnel: [w663 w664] -> w656
                        tunnel: w655 -> [w663 _]
                        frame False {
                        }
                        frame True {
                          n218 = Delete From Array(array=w666, index=w665) -> (array with subset deleted=w664:u32[])  [unwired: 1 in, 1 out]
                        }
                      }
                    }
                  }
                  frame True {
                    # "Atacante já travado"
                  }
                }
                n219 = case shown="True" w646 {
                  tunnel: w645 -> [w669 _]
                  tunnel: [w668 w681] -> w644
                  tunnel: w643 -> [_ w677]
                  tunnel: w642 -> [_ w683]
                  tunnel: w636 -> [_ w680]
                  tunnel: w637 -> [_ w679]
                  tunnel: w641 -> [_ w678]
                  tunnel: w635 -> [_ w676]
                  tunnel: w640 -> [_ w674]
                  tunnel: w639 -> [_ w675]
                  tunnel: w638 -> [_ w673]
                  tunnel: w632 -> [_ w672]
                  tunnel: w631 -> [_ w671]
                  tunnel: w629 -> [_ w670]
                  frame False {
                    # "Personalidade já definida"
                    n220 = Unbundle By Name(w669) -> ("function"=w668:T5)
                  }
                  frame True {
                    # "Id válido para personalidade dinâmica"
                    n221 = Equal?(x=w683, y=w677) -> (x = y?=w682:bool)
                    n222 = case shown="False" w682 {
                      tunnel: [w693 Functions_Enum."Goalie" ("function")] -> w681
                      tunnel: w680 -> [w695 _]
                      tunnel: w679 -> [w694 _]
                      tunnel: w678 -> [w692 _]
                      tunnel: w677 -> [w691 _]
                      tunnel: w676 -> [w690 _]
                      tunnel: w675 -> [w689 _]
                      tunnel: w674 -> [w688 _]
                      tunnel: w673 -> [w687 _]
                      tunnel: w672 -> [w686 _]
                      tunnel: w671 -> [w685 _]
                      tunnel: w670 -> [w684 _]
                      frame False {
                        # "Não é goleiro"
                        n223 = case shown="False" w695 {
                          tunnel: w694 -> [w705 w815]
                          tunnel: [w706 w814] -> w693
                          tunnel: w692 -> [w700 w813]
                          tunnel: w691 -> [w704 w812]
                          tunnel: w690 -> [w702 w811]
                          tunnel: w689 -> [w701 w810]
                          tunnel: w688 -> [w703 _]
                          tunnel: w687 -> [w699 w809]
                          tunnel: w686 -> [w698 w808]
                          tunnel: w685 -> [w697 _]
                          tunnel: w684 -> [w696 _]
                          frame False {
                            # "Attacker ainda não definido"
                            n224 = Index Array(array=w703) -> (element=w708:dbl)  [unwired: 1 in]
                            n225 = Equal?(x=w708, y=w704) -> (x = y?=w707:bool)
                            n226 = case shown="False" w707 {
                              tunnel: [w715 Functions_Enum."Attacker" ("function")] -> w706
                              tunnel: w705 -> [w718 _]
                              tunnel: w704 -> [w717 _]
                              tunnel: w702 -> [w716 _]
                              tunnel: w701 -> [w714 _]
                              tunnel: w700 -> [w713 _]
                              tunnel: w699 -> [w712 _]
                              tunnel: w698 -> [w711 _]
                              tunnel: w697 -> [w710 _]
                              tunnel: w696 -> [w709 _]
                              frame False {
                                # "Robô que está passando pelo código NÃO\né o mais próximo à bola"
                                n227 = case shown="True" w712 {
                                tunnel: w718 -> [_ w728]
                                tunnel: w717 -> [_ w727]
                                tunnel: w716 -> [_ w726]
                                tunnel: [Functions_Enum."Defender" ("function") w725] -> w715
                                tunnel: w714 -> [_ w724]
                                tunnel: w713 -> [_ w723]
                                tunnel: w711 -> [_ w722]
                                tunnel: w710 -> [_ w721]
                                tunnel: w709 -> [_ w720]
                                frame False {
                                # "Não qtdade min p/ Striker"
                                }
                                frame True {
                                # "Tem qtdade min p/ Striker"
                                n228 = case shown="False" w728 {
                                tunnel: w727 -> [w733 w779]
                                tunnel: w726 -> [w732 w778]
                                tunnel: [w736 w781] -> w725
                                tunnel: w724 -> [w735 w782]
                                tunnel: w723 -> [w734 w780]
                                tunnel: w722 -> [w731 w777]
                                tunnel: w721 -> [w730 _]
                                tunnel: w720 -> [w729 _]
                                frame False {
                                # "Striker ainda não definido"
                                n229 = Index Array(array=w732) -> (element=w738:u32)  [unwired: 1 in]
                                n230 = Equal?(x=w738, y=w733) -> (x = y?=w737:bool)
                                n231 = case shown="False" w737 {
                                tunnel: [w745 Functions_Enum."Striker" ("function")] -> w736
                                tunnel: w735 -> [w746 _]
                                tunnel: w734 -> [w744 _]
                                tunnel: w733 -> [w743 _]
                                tunnel: w732 -> [w742 _]
                                tunnel: w731 -> [w741 _]
                                tunnel: w730 -> [w740 _]
                                tunnel: w729 -> [w739 _]
                                frame False {
                                # "Robô que está passando pelo código NÃO\né o de maior id dos não fixados"
                                n232 = case shown="False" w746 {
                                tunnel: [w752 Functions_Enum."Defender" ("function")] -> w745
                                tunnel: w744 -> [w751 _]
                                tunnel: w743 -> [w754 _]
                                tunnel: w742 -> [w753 _]
                                tunnel: w741 -> [w749 _]
                                tunnel: w740 -> [w750 _]
                                tunnel: w739 -> [w747 _]
                                frame False {
                                # "Quando termina o Pass\nState, não precisamos \nmais que o 2nd Stiker \nseja o fixado e o código \nescolhe pelo id."
                                # "2nd Striker NÃO fixado ou fixado com id válido"
                                n233 = case shown="False" w747 {
                                selector: w747 -> [w755 _]
                                tunnel: w749 -> [_ w756]
                                tunnel: [w755 w756] -> w748
                                frame False {
                                }
                                frame True {
                                }
                                }
                                n234 = case shown="True" w748 {
                                tunnel: w754 -> [w760 w772]
                                tunnel: w753 -> [w759 _]
                                tunnel: [w758 w770] -> w752
                                tunnel: w751 -> [w757 _]
                                tunnel: w750 -> [_ w769]
                                frame False {
                                # "2nd Striker não fixado"
                                n235 = case shown="True" w757 {
                                tunnel: w760 -> [_ w766]
                                tunnel: w759 -> [_ w764]
                                tunnel: [Functions_Enum."Defender" ("function") w762] -> w758
                                frame False {
                                # "Quantidade de robôs NÃO\nsuficiente p/ ter 2nd Striker.\nSobra ser defender"
                                }
                                frame True {
                                # "Quantidade de robôs \nsuficiente p/ ter 2nd Striker"
                                n236 = Index Array(array=w764) -> (element #2=w765:u32)  [unwired: 2 in, 1 out]
                                n237 = Equal?(x=w765, y=w766) -> (x = y?=w763:bool)
                                n238 = case shown="True" w763 {
                                tunnel: [Functions_Enum."Defender" ("function") Functions_Enum."2nd Striker" ("function")] -> w762
                                frame False {
                                }
                                frame True {
                                # "Robô que está passando pelo código\né o de segundo maior id dos não fixados"
                                }
                                }
                                }
                                }
                                }
                                frame True {
                                # "2nd Striker travado com id válido"
                                n239 = Equal?(x=w769, y=w772) -> (x = y?=w771:bool)
                                n240 = case shown="True" w771 {
                                tunnel: [Functions_Enum."Defender" ("function") Functions_Enum."2nd Striker" ("function")] -> w770
                                frame False {
                                # "Robô que está passando pelo código NÃO é o fixado como 2nd Striker"
                                }
                                frame True {
                                # "Robô que está passando pelo código é o fixado como 2nd Striker"
                                }
                                }
                                }
                                }
                                }
                                frame True {
                                # "2nd Striker fixado com None"
                                }
                                }
                                }
                                frame True {
                                # "Robô que está passando pelo código\né o de maior id dos não fixados"
                                }
                                }
                                }
                                frame True {
                                # "Striker já travado"
                                n241 = case shown="False" w782 {
                                tunnel: [w784 Functions_Enum."Defender" ("function")] -> w781
                                tunnel: w780 -> [w787 _]
                                tunnel: w779 -> [w786 _]
                                tunnel: w778 -> [w785 _]
                                tunnel: w777 -> [w783 _]
                                frame False {
                                # "2nd Striker NÃO fixado ou fixado com id válido"
                                n242 = case shown="False" w783 {
                                tunnel: w787 -> [w791 _]
                                tunnel: w786 -> [w790 w803]
                                tunnel: w785 -> [w789 _]
                                tunnel: [w788 w800] -> w784
                                frame False {
                                # "2nd Striker não fixado"
                                n243 = case shown="True" w791 {
                                tunnel: w790 -> [_ w797]
                                tunnel: w789 -> [_ w795]
                                tunnel: [Functions_Enum."Defender" ("function") w793] -> w788
                                frame False {
                                # "Quantidade de robôs NÃO\nsuficiente p/ ter 2nd Striker"
                                }
                                frame True {
                                # "Quantidade de robôs \nsuficiente p/ ter 2nd Striker"
                                n244 = Index Array(array=w795) -> (element=w796:u32)  [unwired: 1 in]
                                n245 = Equal?(x=w796, y=w797) -> (x = y?=w794:bool)
                                n246 = case shown="False" w794 {
                                tunnel: [Functions_Enum."Defender" ("function") Functions_Enum."2nd Striker" ("function")] -> w793
                                frame False {
                                # "Robô que está passando pelo código NÃO\né o de maior id dos não fixados"
                                }
                                frame True {
                                # "Robô que está passando pelo código\né o de maior id dos não fixados"
                                }
                                }
                                }
                                }
                                }
                                frame True {
                                # "2nd Striker travado com id válido"
                                n247 = local read "Id 2nd Striker\nPinned"() -> (w802:u32)
                                n248 = Equal?(x=w802, y=w803) -> (x = y?=w801:bool)
                                n249 = case shown="False" w801 {
                                tunnel: [Functions_Enum."Defender" ("function") Functions_Enum."2nd Striker" ("function")] -> w800
                                frame False {
                                # "Robô que está passando no código NÃO é o fixado como 2nd Striker"
                                }
                                frame True {
                                # "Robô que está passando no código é o fixado como 2nd Striker"
                                }
                                }
                                }
                                }
                                }
                                frame True {
                                # "2nd Striker fixado com None"
                                }
                                }
                                }
                                }
                                }
                                }
                              }
                              frame True {
                                # "Robô que está passando pelo código\né o mais próximo à bola"
                              }
                            }
                          }
                          frame True {
                            # "Atacante já travado"
                            n250 = case shown="True" w809 {
                              tunnel: w815 -> [_ w823]
                              tunnel: [Functions_Enum."Defender" ("function") w822] -> w814
                              tunnel: w813 -> [_ w821]
                              tunnel: w812 -> [_ w820]
                              tunnel: w811 -> [_ w819]
                              tunnel: w810 -> [_ w818]
                              tunnel: w808 -> [_ w817]
                              frame False {
                                # "NÃO tem qtdade min p/ Striker"
                              }
                              frame True {
                                # "Tem qtdade min p/ Striker"
                                n251 = case shown="False" w823 {
                                tunnel: [w829 w868] -> w822
                                tunnel: w821 -> [w827 w867]
                                tunnel: w820 -> [w826 w866]
                                tunnel: w819 -> [w825 w865]
                                tunnel: w818 -> [w828 w864]
                                tunnel: w817 -> [w824 w863]
                                frame False {
                                # "Striker ainda não definido"
                                n252 = Index Array(array=w825) -> (element=w831:u32)  [unwired: 1 in]
                                n253 = Equal?(x=w831, y=w826) -> (x = y?=w830:bool)
                                n254 = case shown="False" w830 {
                                tunnel: [w836 Functions_Enum."Striker" ("function")] -> w829
                                tunnel: w828 -> [w837 _]
                                tunnel: w827 -> [w835 _]
                                tunnel: w826 -> [w832 _]
                                tunnel: w825 -> [w834 _]
                                tunnel: w824 -> [w833 _]
                                frame False {
                                # "Robô que está passando pelo código NÃO\né o de maior id dos não fixados"
                                n255 = case shown="False" w837 {
                                tunnel: [w838 Functions_Enum."Defender" ("function")] -> w836
                                tunnel: w835 -> [w840 _]
                                tunnel: w832 -> [w842 _]
                                tunnel: w834 -> [w841 _]
                                tunnel: w833 -> [w839 _]
                                frame False {
                                # "2nd Striker NÃO fixado ou fixado com id válido"
                                n256 = case shown="True" w839 {
                                tunnel: w842 -> [w846 w858]
                                tunnel: w841 -> [w845 _]
                                tunnel: w840 -> [w844 _]
                                tunnel: [w843 w855] -> w838
                                frame False {
                                # "2nd Striker não fixado"
                                n257 = case shown="True" w844 {
                                tunnel: w846 -> [_ w852]
                                tunnel: w845 -> [_ w851]
                                tunnel: [Functions_Enum."Defender" ("function") w848] -> w843
                                frame False {
                                # "Quantidade de robôs NÃO\nsuficiente p/ ter 2nd Striker.\nSobra ser defender"
                                }
                                frame True {
                                # "Quantidade de robôs \nsuficiente p/ ter 2nd Striker"
                                n258 = Index Array(array=w851) -> (element #2=w850:u32)  [unwired: 2 in, 1 out]
                                n259 = Equal?(x=w850, y=w852) -> (x = y?=w849:bool)
                                n260 = case shown="False" w849 {
                                tunnel: [Functions_Enum."Defender" ("function") Functions_Enum."2nd Striker" ("function")] -> w848
                                frame False {
                                }
                                frame True {
                                # "Robô que está passando pelo código\né o de segundo maior id dos não fixados"
                                }
                                }
                                }
                                }
                                }
                                frame True {
                                # "2nd Striker fixado com id válido"
                                n261 = local read "Id 2nd Striker\nPinned"() -> (w857:u32)
                                n262 = Equal?(x=w857, y=w858) -> (x = y?=w856:bool)
                                n263 = case shown="True" w856 {
                                tunnel: [Functions_Enum."Defender" ("function") Functions_Enum."2nd Striker" ("function")] -> w855
                                frame False {
                                # "Robô que está passando pelo código NÃO é o 2nd Striker fixado no pinned"
                                }
                                frame True {
                                # "Robô que está passando pelo código é o 2nd Striker fixado no pinned"
                                }
                                }
                                }
                                }
                                }
                                frame True {
                                # "2nd Striker fixado com id inválido (None)"
                                }
                                }
                                }
                                frame True {
                                # "Robô que está passando pelo código\né o de maior id dos não fixados"
                                }
                                }
                                }
                                frame True {
                                # "Striker já travado"
                                n264 = case shown="False" w864 {
                                tunnel: [w872 Functions_Enum."Defender" ("function")] -> w868
                                tunnel: w867 -> [w873 _]
                                tunnel: w866 -> [w871 _]
                                tunnel: w865 -> [w870 _]
                                tunnel: w863 -> [w869 _]
                                frame False {
                                # "2nd Striker não fixado ou fixado com id válido"
                                n265 = case shown="True" w869 {
                                tunnel: w873 -> [w877 _]
                                tunnel: [w876 w886] -> w872
                                tunnel: w871 -> [w875 w889]
                                tunnel: w870 -> [w874 _]
                                frame False {
                                # "2nd Striker não fixado"
                                n266 = case shown="False" w877 {
                                tunnel: [Functions_Enum."Defender" ("function") w879] -> w876
                                tunnel: w875 -> [_ w883]
                                tunnel: w874 -> [_ w882]
                                frame False {
                                # "Quantidade de robôs NÃO\nsuficiente p/ ter 2nd Striker.\nSobra ser defender"
                                }
                                frame True {
                                # "Quantidade de robôs \nsuficiente p/ ter 2nd Striker"
                                n267 = Index Array(array=w882) -> (element=w881:u32)  [unwired: 1 in]
                                n268 = Equal?(x=w881, y=w883) -> (x = y?=w880:bool)
                                n269 = case shown="False" w880 {
                                tunnel: [Functions_Enum."Defender" ("function") Functions_Enum."2nd Striker" ("function")] -> w879
                                frame False {
                                }
                                frame True {
                                # "Robô que está passando pelo código\né o de maior id dos não fixados"
                                }
                                }
                                }
                                }
                                }
                                frame True {
                                # "2nd Striker fixado com id válido"
                                n270 = local read "Id 2nd Striker\nPinned"() -> (w888:u32)
                                n271 = Equal?(x=w888, y=w889) -> (x = y?=w887:bool)
                                n272 = case shown="True" w887 {
                                tunnel: [Functions_Enum."Defender" ("function") Functions_Enum."2nd Striker" ("function")] -> w886
                                frame False {
                                # "Robô que está passando no código NÃO é o robô fixado, no pinned, para ser 2nd Striker"
                                }
                                frame True {
                                # "Robô que está passando no código é o robô fixado, no pinned, para ser 2nd Striker"
                                }
                                }
                                }
                                }
                                }
                                frame True {
                                # "2nd Striker fixado com id inválido (None)"
                                }
                                }
                                }
                                }
                              }
                            }
                          }
                        }
                      }
                      frame True {
                        # "É goleiro"
                      }
                    }
                  }
                }
              }
              frame True {
                # "Após ter iniciado o evento de passe,\nAttacker já tocou a bola mas ainda \nnão acabou o pass state."
                n273 = Index Array(array=w941, index=w940) -> (element=w939:T4)
                n274 = Unbundle By Name(w939) -> ("function"=w938:T5)
              }
            }
            n275 = Bundle By Name(cluster=w616, "function"=w624) -> (w626:T4)
          }
        }
      }
    }
  }
  n276 = feedback-in #2(w43) -> ()
  n277 = feedback-in #3(w35) -> ()
  n278 = Unbundle By Name(w103) -> ("Events.Kick"=w112:bool, "balls"=w121:T9[])
  n279 = for {
    shift-right: [w955] -> w9
    shift-left: _ -> [w953]
    tunnel: w35 -> [w952] mode=indexing
    n280 = Unbundle By Name(w952) -> ("id"=w954:u32, "function"=w951:T5)
    n281 = Equal?(x=w951, y=Functions_Enum."Striker") -> (x = y?=w950:bool)
    n282 = case shown="True" w950 {
      tunnel: [w957 w958] -> w955
      tunnel: w954 -> [_ w958]
      tunnel: w953 -> [w957 _]
      frame False {
      }
      frame True {
      }
    }
  }
  n283 = for {
    tunnel: w35 -> [w965] mode=indexing
    shift-right: [w959] -> w37
    shift-left: u32[] [] -> [w961]
    n284 = Unbundle By Name(w965) -> ("id"=w960:u32, "function"=w964:T5)
    n285 = Equal?(x=w964, y=Functions_Enum."Defender") -> (x = y?=w962:bool)
    n286 = case shown="True" w962 {
      tunnel: w961 -> [w966 w969]
      tunnel: w960 -> [_ w968]
      tunnel: [w966 w967] -> w959
      frame False {
      }
      frame True {
        n287 = Insert Into Array(array=w969, new element=w968) -> (w967:u32[])  [unwired: 1 in]
      }
    }
  }
  n288 = Index Array(array=w121) -> (element=w120:T9)  [unwired: 1 in]
  n289 = Unbundle By Name(w120) -> ("Vel_x"=w110:dbl, "Vel_y"=w109:dbl, "x"=w119:dbl, "y"=w118:dbl)
  n290 = Build Array(w110, w109) -> (w108:dbl[])
  n291 = Build Array(w119, w118) -> (w33:dbl[])
  n292 = case shown="False" w112 {
    selector: w112 -> [_ w979]
    tunnel: [w971 w979] -> w113
    tunnel: w111 -> [w970 _]
    tunnel: w108 -> [w977 _]
    tunnel: [w973 FALSE] -> _
    frame False {
      n293 = call "Modulo.vi"("2D vector"=w977) -> ("Modulo"=w976:dbl)  [unwired: 10 in]
      n294 = Less?(x=w976, y=0.01) -> (x < y?=w974:bool)
      n295 = And(x=w974, y=w970) -> (x .and. y?=w973:bool)
      n296 = Select(t=FALSE ("Kick"), s=w973, f=w970) -> (s? t:f=w971:bool)
    }
    frame True {
    }
  }
  n297 = feedback-in #4(w113) -> ()
  n298 = Array Max & Min(array=w37) -> (max value=w14:u32)  [unwired: 3 out]
  n299 = case shown="False" w11 {
    tunnel: [u32 42 ("id") w981] -> w10
    tunnel: w9 -> [_ w981]
    frame False {
      # "Strk None"
    }
    frame True {
      # "Strk existe"
    }
  }
  n300 = feedback-in #5(w3) -> ()
  n301 = Not Equal?(x=w3, y=w2) -> (x != y?=w1:bool)
  n302 = Not(x=w1) -> (.not. x?=w8:bool)
  n303 = Compound Arithmetic op=AND(w6, w5, w8) -> (w4:bool)
  n304 = Bundle By Name(cluster=w103, "our_robots"=w35) -> (w64:T3)
  n305 = case shown="False" w16 {
    tunnel: w15 -> [_ w983]
    tunnel: [w982 w983] -> w13
    tunnel: w14 -> [w982 _]
    frame False {
    }
    frame True {
      # "2nd Striker pinned com id válido"
    }
  }
  n306 = case shown="True" w23 {
    tunnel: [w985 w987] -> w39
    tunnel: w10 -> [w985 _]
    tunnel: w40 -> [_ w987]
    tunnel: w13 -> [w984 _]
    tunnel: [w984 w986] -> w34
    tunnel: w36 -> [_ w986]
    frame False {
      # "Estado normal"
    }
    frame True {
      # "Estado de passe"
    }
  }
  n307 = for {
    tunnel: w35 -> [w997] mode=indexing
    tunnel: w33 -> [w993]
    shift-right: [w992] -> w107
    shift-left: FALSE -> [w991]
    tunnel: w39 -> [w990]
    n308 = Unbundle By Name(w997) -> ("x"=w996:dbl, "y"=w995:dbl, "id"=w989:u32)
    n309 = Equal?(x=w989, y=w990) -> (x = y?=w988:bool)
    n310 = Build Array(w996, w995) -> (w994:dbl[])
    n311 = case shown="True" w988 {
      tunnel: w994 -> [_ w1003]
      tunnel: w993 -> [_ w1004]
      tunnel: [w998 w999] -> w992
      tunnel: w991 -> [w998 _]
      frame False {
      }
      frame True {
        n312 = Subtract(x=w1004, y=w1003) -> (x-y=w1002:dbl[])
        n313 = call "Modulo.vi"("2D vector"=w1002) -> ("Modulo"=w1001:dbl)  [unwired: 10 in]
        n314 = Less?(x=w1001, y=200.0) -> (x < y?=w999:bool)
      }
    }
  }
  n315 = for {
    tunnel: w35 -> [w1014] mode=indexing
    tunnel: w34 -> [w1012]
    tunnel: w33 -> [w1007]
    shift-right: [w1006] -> w31
    shift-left: FALSE -> [w1005]
    n316 = Unbundle By Name(w1014) -> ("x"=w1010:dbl, "y"=w1009:dbl, "id"=w1013:u32)
    n317 = Equal?(x=w1013, y=w1012) -> (x = y?=w1011:bool)
    n318 = Build Array(w1010, w1009) -> (w1008:dbl[])
    n319 = case shown="True" w1011 {
      tunnel: w1008 -> [_ w1021]
      tunnel: w1007 -> [_ w1020]
      tunnel: [w1015 w1016] -> w1006
      tunnel: w1005 -> [w1015 _]
      frame False {
      }
      frame True {
        n320 = Subtract(x=w1021, y=w1020) -> (x-y=w1019:dbl[])
        n321 = call "Modulo.vi"("2D vector"=w1019) -> ("Modulo"=w1018:dbl)  [unwired: 10 in]
        n322 = Less?(x=w1018, y=200.0) -> (x < y?=w1016:bool)
      }
    }
  }
  n323 = feedback-in #6(w39) -> ()
  n324 = feedback-in #7(w34) -> ()
  n325 = Compound Arithmetic op=OR(w31, FALSE ("value"), w107) -> (w106:bool)
  n326 = feedback-in #8(w106) -> ()
  n327 = feedback #11(w64) -> (w102:T3)
  n328 = case shown="True" w4 {
    tunnel: w102 -> [_ w1028]
    tunnel: [w1022 w1023] -> w96
    tunnel: w64 -> [w1022 w1024]
    frame False {
    }
    frame True {
      n329 = Unbundle By Name(w1024) -> ("our_robots"=w1026:T4[])
      n330 = Unbundle By Name(w1028) -> ("our_robots"=w1027:T4[])
      n331 = for {
        tunnel: w1027 -> [w1031] mode=indexing
        tunnel: w1026 -> [w1032] mode=indexing
        tunnel: [w1029] -> w1025 mode=indexing
        n332 = Unbundle By Name(w1031) -> ("function"=w1030:T5)
        n333 = Bundle By Name(cluster=w1032, "function"=w1030) -> (w1029:T4)
      }
      n334 = Bundle By Name(cluster=w1024, "our_robots"=w1025) -> (w1023:T3)
    }
  }
  n335 = Unbundle By Name(w102) -> ("our_robots"=w100:T4[])
  n336 = Array Size(array=w100) -> (size(s)=w98:i32)
  n337 = Unbundle By Name(w64) -> ("our_robots"=w101:T4[])
  n338 = Array Size(array=w101) -> (size(s)=w99:i32)
  n339 = Not Equal?(x=w98, y=w99) -> (x != y?=w97:bool)
  n340 = case shown="False" w97 {
    tunnel: w96 -> [w1033 _]
    tunnel: [w1033 w1034] -> w95
    tunnel: w64 -> [_ w1034]
    frame False {
    }
    frame True {
    }
  }
  n341 = First Call?() -> (First Call?: T/F=w94:bool)
  n342 = case shown="True" w94 {
    tunnel: [w1035 w1036] -> w86
    tunnel: w95 -> [w1035 _]
    tunnel: w64 -> [_ w1036]
    frame False {
    }
    frame True {
    }
  }
  n343 = feedback-in #12("Pinned") -> ()
  n344 = feedback #12() -> (w93:T1)  [unwired: 1 in]
  n345 = Unbundle By Name("Pinned") -> ("Attc"=w92:T2, "Strk"=w90:T2, "Def"=w77:T2[])
  n346 = Unbundle By Name(w93) -> ("Attc"=w91:T2, "Strk"=w89:T2, "Def"=w78:T2[])
  n347 = Not Equal?(x=w92, y=w91) -> (x != y?=w87:bool)
  n348 = Not Equal?(x=w90, y=w89) -> (x != y?=w88:bool)
  n349 = Not Equal?(x=w77, y=w78) -> (x != y?=w76:bool[])
  n350 = Or Array Elements(Boolean array=w76) -> (logical OR=w75:bool)
  n351 = Compound Arithmetic op=OR(w87, w88, w75) -> (w85:bool)
  n352 = case shown="True" w85 {
    tunnel: w86 -> [w1037 _]
    tunnel: [w1037 w1038] -> w82
    tunnel: w64 -> [_ w1038]
    frame False {
    }
    frame True {
    }
  }
  n353 = feedback #13() -> (w84:bool)  [unwired: 1 in]
  n354 = feedback-in #13("Modo Teste ?") -> ()
  n355 = Not Equal?(x=w84, y="Modo Teste ?") -> (x != y?=w83:bool)
  n356 = case shown="False" w83 {
    tunnel: w64 -> [_ w1040]
    tunnel: [w1039 w1040] -> w63
    tunnel: w82 -> [w1039 _]
    frame False {
    }
    frame True {
    }
  }
  n357 = Unbundle By Name("input cluster") -> ("IA Judge.command enum"=w69:T12)
  n358 = Equal?(x=w69, y=Command_Enum."Prepare Penalty Enemy" ("IA Judge.command enum")) -> (x = y?=w67:bool)
  n359 = Equal?(x=w69, y=Command_Enum."PPE Normal Start" ("IA Judge.command enum")) -> (x = y?=w66:bool)
  n360 = Or(x=w67, y=w66) -> (x .or. y?=w65:bool)
  n361 = case shown="True" w65 {
    tunnel: w64 -> [_ w1042]
    tunnel: [w1041 w1042] -> w62
    tunnel: w63 -> [w1041 _]
    frame False {
    }
    frame True {
    }
  }
  "output cluster" <- w62
  n362 = feedback-in #11(w62) -> ()
